vi "full screen.vi"() -> ()   [LabVIEW 2011]
uses:
  <vilib>/Utility/miscctls.llb/LVRectTypeDef.ctl
panel:
  out "Display:Primary Workspace":T1
  in  "stop":bool
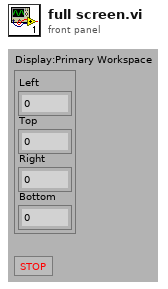
[diagram p1: front panel]
types:
  T1 = typedef "LVRectTypeDef.ctl" = cluster{"Left":i16, "Top":i16, "Right":i16, "Bottom":i16}
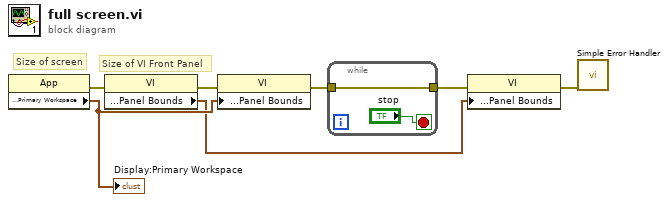
[diagram p0: block diagram]
diagram:
  # "Size of VI Front Panel"
  # "Size of screen"
  n1 = property class="App"() -> (error out=w5:errorcluster, "Display:Primary Workspace"=w7:T1)  [unwired: 2 in, 1 out]
  "Display:Primary Workspace" <- w7
  n2 = property class="VI"(error in=w5) -> (error out=w4:errorcluster, "Front Panel Window:Panel Bounds"=w2:T1)  [unwired: 1 in, 1 out]
  n3 = property class="VI"(error in=w4, "Front Panel Window:Panel Bounds"=w7) -> (error out=w6:errorcluster)  [unwired: 1 in, 1 out]
  n4 = while {
    tunnel: w6 -> [w8]
    tunnel: [w8] -> w3
    stop <- "stop" stop-if-true
  }
  n5 = property class="VI"(error in=w3, "Front Panel Window:Panel Bounds"=w2) -> (error out=w1:errorcluster)  [unwired: 1 in, 1 out]
  n6 = call <vilib>:"Simple Error Handler.vi"("error in (no error)"=w1) -> ()  [unwired: 1 in, 8 out]
